vi "Reinitialize.vi"(8 "error in (no error)":errorcluster, 11 "SOL MS in":refnum<class "PL SOL Instruments MS.lvclass">) -> (0 "error out":errorcluster, 3 "SOL MS out":refnum<class "PL SOL Instruments MS.lvclass">)   [LabVIEW 2015, in "PL SOL Instruments MS.lvclass"]
doc: "Reinitializes connection to device based on previously specified settings."
uses:
  PL SOL Instruments MS.lvclass
  PL SOL Instruments MS.lvclass/PL SOL Instruments MS.ctl
  <vilib>/Instr/_visa.llb/VISA Configure Serial Port (Instr).vi
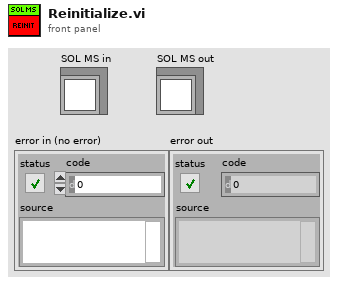
[diagram p1: front panel]
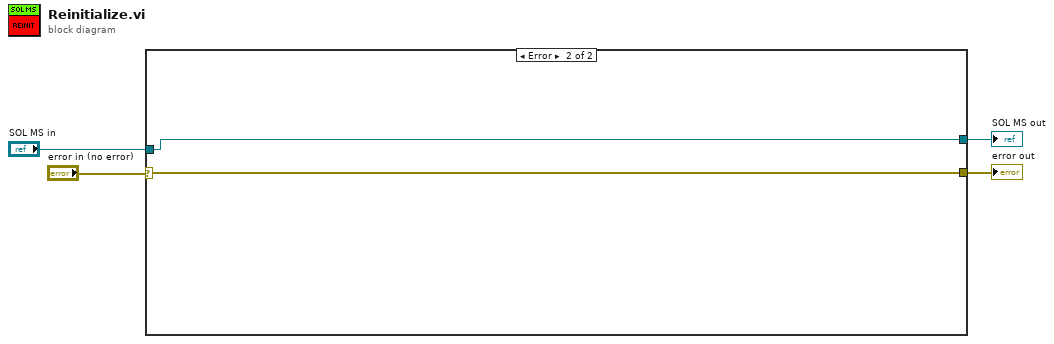
[diagram p0: block diagram]
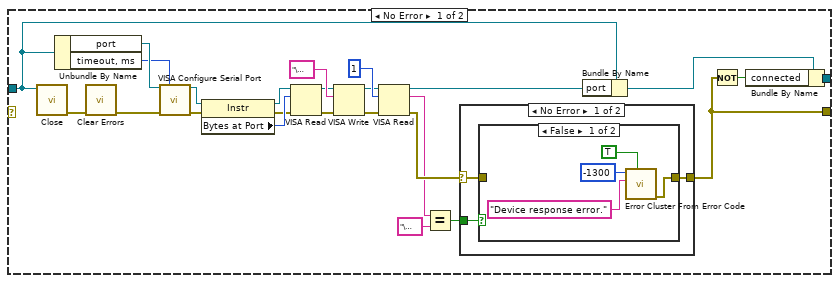
[diagram p2: hidden frame]
diagram:
  n1 = case shown="Error" "error in (no error)" {
    selector: "error in (no error)" -> [_ w39]
    tunnel: "SOL MS in" -> [w29 w40]
    tunnel: [w26 w40] -> w3
    tunnel: [w13 w39] -> w2
    frame No Error {
      n2 = call "Close.vi"("SOL MS in"=w29) -> ("error out"=w6:errorcluster)  [unwired: 10 in]
      n3 = Unbundle By Name(w29) -> ("port"=w25:refnum<visa-resource-name>, "timeout, ms"=w20:u32)
      n4 = call <vilib>:"Clear Errors.vi"("error in (no error)"=w6) -> ("error out"=w5:errorcluster)  [unwired: 5 in, 1 out]
      n5 = call-poly "VISA Configure Serial Port"("VISA resource name"=w25, "timeout (10sec)"=w20, "error in (no error)"=w5) -> ("VISA resource name out"=w21:refnum<visa-resource-name>, "error out"=w19:errorcluster)  [unwired: 11 in]
      n6 = property class="Instr"(reference=w21, error in=w19) -> (reference out=w8:refnum<visa-resource-name>, error out=w7:errorcluster, "Bytes at Port"=w9:u32)
      n7 = VISA Read(VISA resource name=w8, byte count=w9, error in (no error)=w7) -> (VISA resource name out=w10:refnum<visa-resource-name>, error out=w11:errorcluster)  [unwired: 2 out]
      n8 = VISA Write(VISA resource name=w10, write buffer="\u0006" ("command"), error in (no error)=w11) -> (VISA resource name out=w17:refnum<visa-resource-name>, error out=w16:errorcluster)  [unwired: 1 out]
      n9 = VISA Read(VISA resource name=w17, byte count=u32 1, error in (no error)=w16) -> (VISA resource name out=w15:refnum<visa-resource-name>, read buffer=w12:string, error out=w14:errorcluster)  [unwired: 1 out]
      n10 = Equal?(x=w12, y="\u0006" ("command")) -> (x = y?=w23:bool)
      n11 = case shown="No Error" w14 {
        selector: w14 -> [w31 w38]
        tunnel: w23 -> [w32 _]
        tunnel: [w30 w38] -> w13
        frame No Error {
          n12 = case shown="False" w32 {
            tunnel: w31 -> [_ w37]
            tunnel: [w34 w37] -> w30
            frame False {
              n13 = call <vilib>:"Error Cluster From Error Code.vi"("show call chain? (False)"=TRUE, "error message (\"\")"="Device response error." ("error message (\"\")"), "error code (0)"=-1300) -> ("error out"=w34:errorcluster)  [unwired: 6 in]
            }
            frame True {
            }
          }
        }
        frame Error {
        }
      }
      n14 = Bundle By Name(cluster=w29, "port"=w15) -> (w28:refnum<class "PL SOL Instruments MS.lvclass">)
      n15 = Not(x=w13) -> (.not. x?=w27:bool)
      n16 = Bundle By Name(cluster=w28, "connected"=w27) -> (w26:refnum<class "PL SOL Instruments MS.lvclass">)
    }
    frame Error {
    }
  }
  "SOL MS out" <- w3
  "error out" <- w2
